vi "Remove Channel.vi"(6 "Index":i32, 7 "Display State In":T1={"Current Channels Info"=[], "Help Prefix"="", "Max Display Size"=8, "Max Size"=0, "Show Buttons"=TRUE, "Data Valid"=refnum, "Show Range"=FALSE, "Range Items"=[], "Range Index"=[]}, 11 "Channels In":T4) -> (3 "Channels Out":T4, 5 "Display State Out":T1={"Current Channels Info"=[], "Help Prefix"="", "Max Display Size"=8, "Max Size"=0, "Show Buttons"=TRUE, "Data Valid"=refnum, "Show Range"=FALSE, "Range Items"=[], "Range Index"=[]})   [LabVIEW 2021, in "myRIO Channel List.xctl"]
uses:
  <vilib>/myRIO/Common/Express VI Framework/xctls/myRIO Channel List/myRIO Channel List.xctl
  <vilib>/myRIO/Common/Express VI Framework/xctls/myRIO Channel List/Data.ctl
  <vilib>/myRIO/Common/Express VI Framework/xctls/myRIO Channel List/typedefs/Channel Data.ctl
  <vilib>/myRIO/Common/Express VI Framework/xctls/myRIO Channel List/typedefs/Remove Channel.ctl
  <vilib>/myRIO/Common/Express VI Framework/xctls/myRIO Channel List/State.ctl
  <vilib>/myRIO/Common/Profile Manager Framework/typedefs/Channel Info.ctl
  <vilib>/myRIO/Common/Express VI Framework/typedefs/Data Validate Ref.ctl
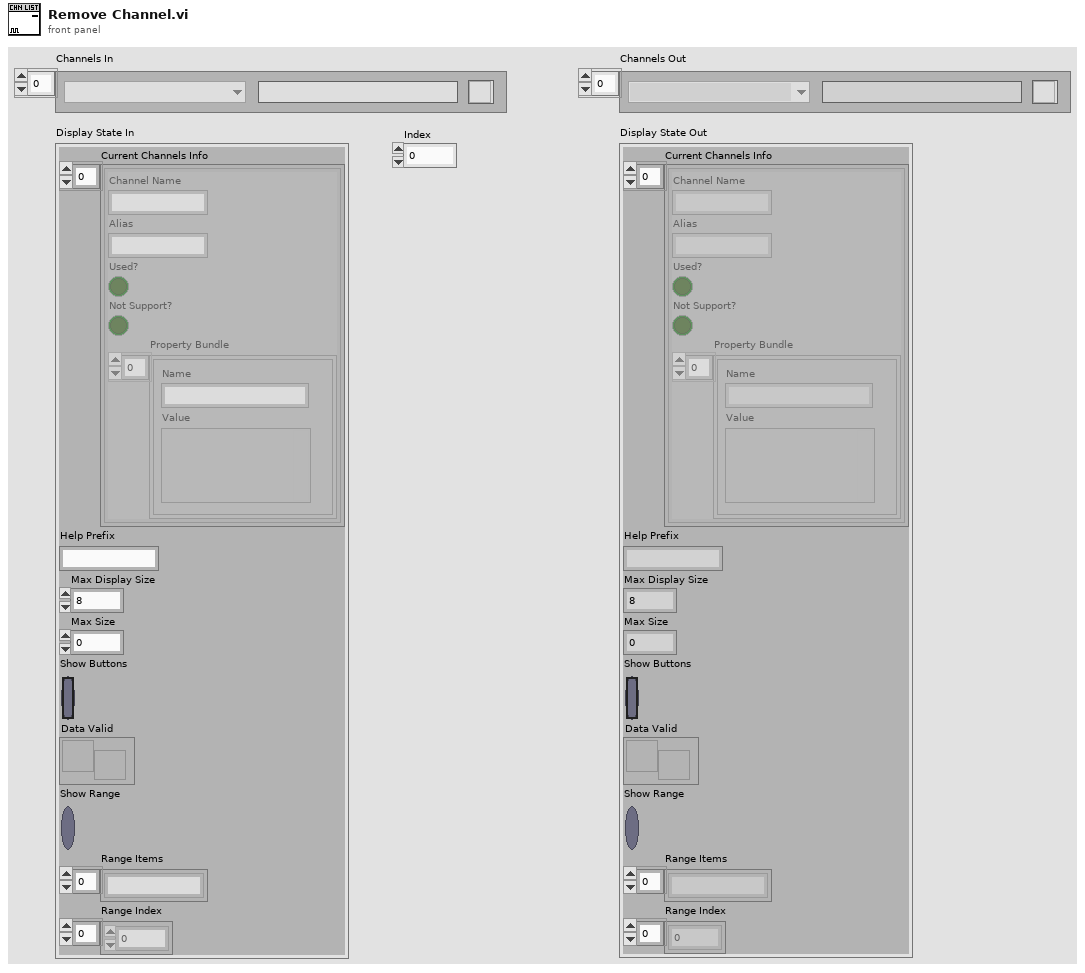
[diagram p1: front panel]
types:
  T1 = typedef "myRIO Channel List.xctl/State.ctl" = cluster{"Current Channels Info":T2[], "Help Prefix":string, "Max Display Size":i32, "Max Size":i32, "Show Buttons":bool, "Data Valid":T3, "Show Range":bool, "Range Items":string[], "Range Index":i32[]}
  T2 = typedef "Channel Info.ctl" = cluster{"Channel Name":string, "Alias":string, "Used?":bool, "Not Support?":bool, "Property Bundle":cluster{"Name":string, "Value":variant}[]}
  T3 = typedef "Data Validate Ref.ctl" = refnum<user-event>
  T4 = typedef "myRIO Channel List.xctl/Data.ctl" = T5[]
  T5 = typedef "myRIO Channel List.xctl/Channel Data.ctl" = cluster{"Channel Name":u16, "Channel Alias":string, "Remove Channel":T6, "Index":i32}
  T6 = typedef "myRIO Channel List.xctl/Remove Channel.ctl" = bool
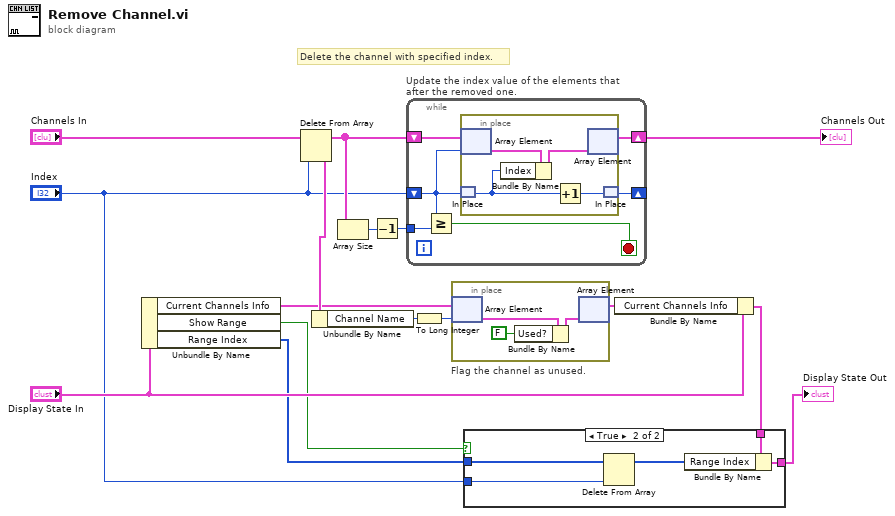
[diagram p0: block diagram]
diagram:
  # "Delete the channel with specified index."
  n1 = Unbundle By Name("Display State In") -> ("Current Channels Info"=w8:T2[], "Show Range"=w2:bool, "Range Index"=w4:i32[])
  n2 = Delete From Array(array="Channels In", index="Index") -> (deleted portion=w11:T5, array with subset deleted=w15:T4)  [unwired: 1 in]
  n3 = Unbundle By Name(w11) -> ("Channel Name"=w10:u16)
  n4 = Array Size(array=w15) -> (size(s)=w14:i32)
  n5 = Decrement(x=w14) -> (x-1=w13:i32)
  n6 = while "Update the index value of the elements that after the removed one." {
    tunnel: w13 -> [w19]
    shift-right: [w21] -> _
    shift-left: "Index" -> [w18]
    shift-right: [w20] -> w12
    shift-left: w15 -> [w22]
    stop <- w17 stop-if-true
    n7 = Greater Or Equal?(x=w18, y=w19) -> (x >= y?=w17:bool)
    n8 = in-place {
      n9 = in-place-array #1(w22, w18) -> (w26:T5)
      n10 = in-place-match #2(w18) -> (w24:i32)
      n11 = Bundle By Name(cluster=w26, "Index"=w24) -> (w25:T5)
      n12 = Increment(x=w24) -> (x+1=w23:i32)
      n13 = in-place-array #1(w25) -> (w20:T4)  [unwired: 1 out]
      n14 = in-place-match #2(w23) -> (w21:i32)
    }
  }
  "Channels Out" <- w12
  n15 = To Long Integer(number=w10) -> (32bit integer=w9:i32)
  n16 = in-place "Flag the channel as unused." {
    n17 = in-place-array #3(w8, w9) -> (w29:T2)
    n18 = Bundle By Name(cluster=w29, "Used?"=FALSE) -> (w28:T2)
    n19 = in-place-array #3(w28) -> (w6:T2[])  [unwired: 1 out]
  }
  n20 = Bundle By Name(cluster="Display State In", "Current Channels Info"=w6) -> (w3:T1)
  n21 = case shown="True" w2 {
    tunnel: "Index" -> [_ w35]
    tunnel: w4 -> [_ w34]
    tunnel: w3 -> [w30 w33]
    tunnel: [w30 w31] -> w1
    frame False {
    }
    frame True {
      n22 = Delete From Array(array=w34, index=w35) -> (array with subset deleted=w32:i32[])  [unwired: 1 in, 1 out]
      n23 = Bundle By Name(cluster=w33, "Range Index"=w32) -> (w31:T1)
    }
  }
  "Display State Out" <- w1
